vi "2_2.vi"() -> ()   [LabVIEW 2010]
uses:
  <vilib>/Analysis/Matrix/Datatypes/RealMatrix.ctl
  <vilib>/Analysis/7linalg.llb/Solve Linear Equations (single right hand).vi
  <vilib>/Analysis/NI_AALPro.lvlib
  <vilib>/Analysis/Matrix/NI_Matrix.lvlib
panel:
  out "Solution Vector":dbl[](array[numeric]) format="%.2f"
  in  "Input Matrix":T1
  in  "Known Vector":dbl[](array[numeric]) format="%.2f"
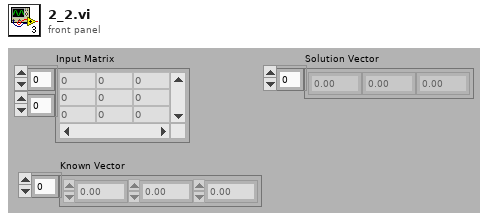
[diagram p1: front panel]
types:
  T1 = typedef "NI_Matrix.lvlib/RealMatrix.ctl" = dbl[][]
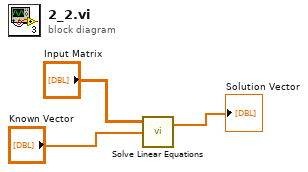
[diagram p0: block diagram]
diagram:
  n1 = call-poly <vilib>:"Solve Linear Equations.vi"("Known Vector"="Known Vector", "Input Matrix"="Input Matrix") -> ("Solution Vector"=→"Solution Vector":dbl[])  [unwired: 1 in, 1 out]
